vi "get_objects.vi"(0 "HGF_FGV_Select":refnum<class "HGF_FGV_Selection.lvclass">, 5 "error in (no error)":errorcluster) -> (14 "dup HGF_FGV_Select":refnum<class "HGF_FGV_Selection.lvclass">, 16 "Objects":refnum<class>[](array[class]), 17 "indexArray":u32[](array[numeric]), 19 "error out":errorcluster)   [LabVIEW 2012, in "HGF_FGV.lvlib" / "HGF_FGV_Selection.lvclass"]
doc: "Returns the indexed objects."
uses:
  HGF_FGV_Selection.lvclass
  HGF_FGV_Selection.lvclass/HGF_FGV_Selection.ctl
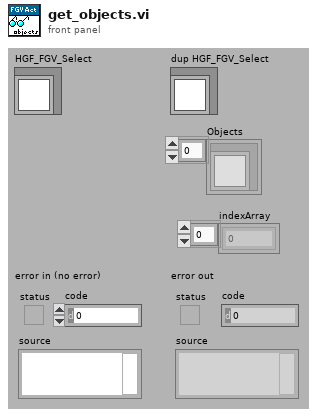
[diagram p1: front panel]
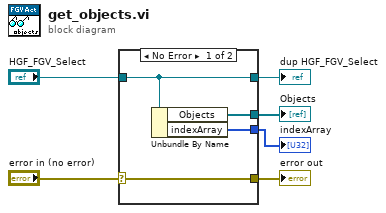
[diagram p0: block diagram]
diagram:
  n1 = case shown="No Error" "error in (no error)" {
    selector: "error in (no error)" -> [w10 w11]
    tunnel: [w10 w11] -> w5
    tunnel: [w9 w12] -> w3
    tunnel: "HGF_FGV_Select" -> [w9 w12]
    tunnel: [w8 _] -> w2
    tunnel: [w7 _] -> w1
    frame No Error {
      n2 = Unbundle By Name(w9) -> ("Objects"=w8:refnum<class>[], "indexArray"=w7:u32[])
    }
    frame Error {
    }
  }
  "error out" <- w5
  "dup HGF_FGV_Select" <- w3
  "Objects" <- w2
  "indexArray" <- w1
